vi "Get Attributes.vi"(8 "error in (no error)":errorcluster, 11 "For Loop Dialog in":refnum<class "Conditional Dialog.lvclass">) -> (0 "error out":errorcluster, 3 "For Loop Dialog out":refnum<class "Conditional Dialog.lvclass">)   [LabVIEW 2017, in "Conditional Dialog.lvclass"]
uses:
  Conditional Dialog.lvclass
  D:/Test-executive-builder/Source/Test Executive Builder Dialogs/ITest Executive Builder Dialog/ITest Executive Builder Dialog.lvclass
  ITest Executive Builder Dialog/ITest Executive Builder Dialog.lvclass/ITest Executive Builder Dialog.ctl
  Conditional Dialog.lvclass/Conditional Dialog.ctl
  210526c6-8347-4f83-98d4-bf6ff259764b.vi
  6281bc39-4b1f-4fa0-b6e5-3275a081bde5.vi
  37054371-845d-43d0-a581-1ea5269a3f09.vi
  <vilib>/Utility/error.llb/Clear Errors.vi
  <vilib>/gpm_packages/@cs/test-executive/Source/Test Executive/ITestExecutive/ITest Executive.lvclass
  Data Type Handler/Test Executive Builder Data Type Handler.lvclass
  ITest Executive Builder Dialog/ITest Executive Builder Dialog.lvclass
  <vilib>/gpm_packages/@cs/test-executive/Source/Test Executive/TestExecutive Ref/TestExecutive Ref.lvclass
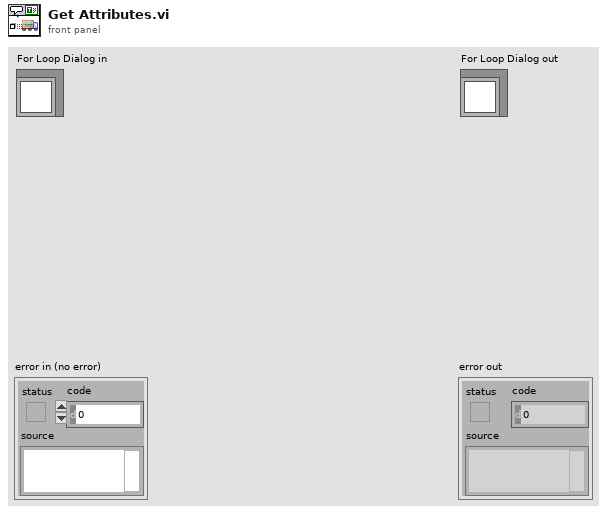
[diagram p1: front panel]
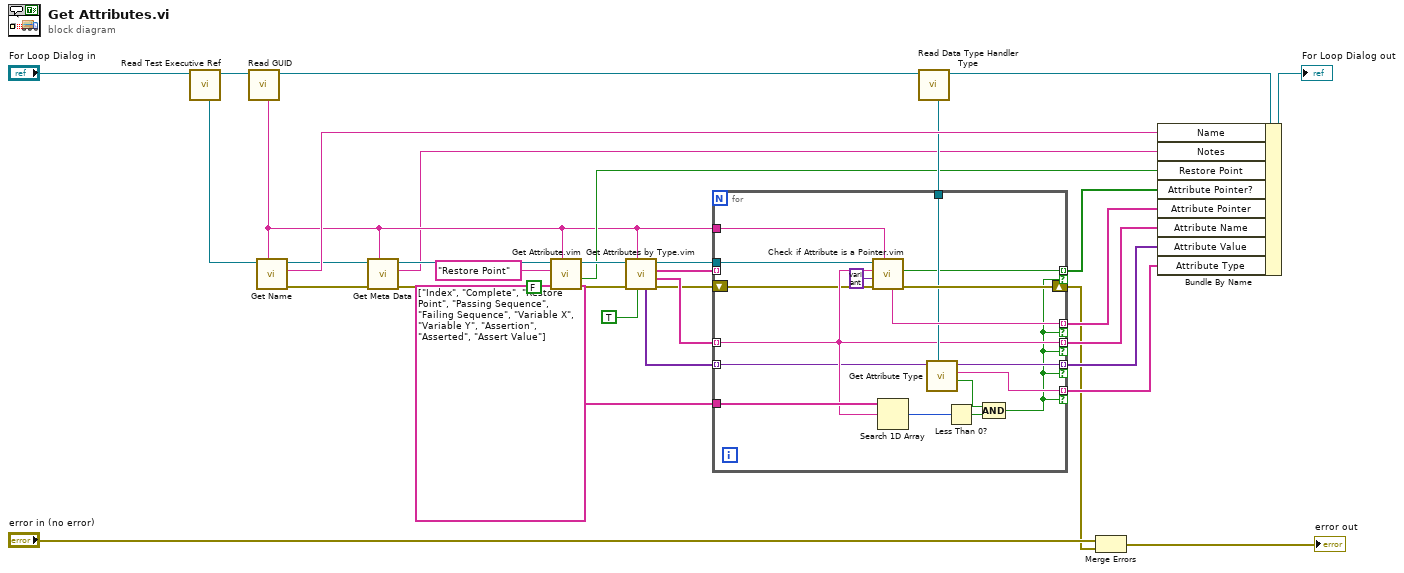
[diagram p0: block diagram]
diagram:
  n1 = call "Read Test Executive Ref.vi"("ITest Executive Builder Dialog in"="For Loop Dialog in") -> ("ITest Executive Builder Dialog out"=w33:refnum<class "Conditional Dialog.lvclass">, "Test Executive Ref"=w30:refnum<data-value>)  [unwired: 9 in]
  n2 = call "Read GUID.vi"("ITest Executive Builder Dialog in"=w33) -> ("ITest Executive Builder Dialog out"=w17:refnum<class "Conditional Dialog.lvclass">, "GUID"=w2:string)  [unwired: 9 in]
  n3 = call <vilib>:"Get Name.vi"("Unique ID"=w2, "Test Executive Ref"=w30) -> ("error out"=w4:errorcluster, "Name"=w32:string, "Test Executive Ref out"=w6:refnum<data-value>)  [unwired: 5 in, 2 out]
  n4 = call <vilib>:"Get Meta Data.vi"("Unique ID"=w2, "error in (no error)"=w4, "Test Executive Ref"=w6) -> ("error out"=w3:errorcluster, "Meta Data"=w1:string, "Test Executive Ref out"=w5:refnum<data-value>)  [unwired: 6 in]
  n5 = call "Get Attribute.vim"("ID"=w2, "error in (no error)"=w3, "Type"=FALSE, "Attribute Name"="Restore Point", "Test Executive Ref"=w5) -> ("error out"=w24:errorcluster, "Attribute"=w13:bool, "Test Executive Ref out"=w25:refnum<data-value>)  [unwired: 2 in, 2 out]
  n6 = call "Get Attributes by Type.vim"("Recurse Up List (Default=True)"=TRUE, "ID"=w2, "error in (no error)"=w24, "Test Executive Ref"=w25) -> ("error out"=w19:errorcluster, "Names"=w20:string[], "IDs"=w21:string[], "Test Executive Ref out"=w22:refnum<data-value>, "Attributes"=w18:variant[])  [unwired: 3 in]
  n7 = call "Read Data Type Handler Type.vi"("ITest Executive Builder Dialog in"=w17) -> ("ITest Executive Builder Dialog out"=w16:refnum<class "Conditional Dialog.lvclass">, "Data Type Handler"=w15:refnum<class "Test Executive Builder Data Type Handler.lvclass">)  [unwired: 9 in]
  n8 = for {
    tunnel: w22 -> [w37]
    tunnel: w21 -> [_] mode=indexing
    tunnel: w20 -> [w40] mode=indexing
    shift-right: [w50] -> w7
    shift-left: w19 -> [w36]
    tunnel: w2 -> [w41]
    tunnel: w18 -> [w39] mode=indexing
    tunnel: [w35] -> w12 mode=indexing if=w38
    tunnel: [w49] -> w11 mode=indexing if=w38
    tunnel: [w40] -> w10 mode=indexing if=w38
    tunnel: w15 -> [w48]
    tunnel: [w46] -> w8 mode=indexing if=w38
    tunnel: [w45] -> w9 mode=indexing if=w38
    tunnel: string[] ["Index", "Complete", "Restore Point", "Passing Sequence", "Failing Sequence", "Variable X", "Variable Y", "Assertion", "Asserted", "Assert Value"] -> [w44]
    n9 = call "Check if Attribute is a Pointer.vim"("ID"=w41, "error in (no error)"=w36, "Type"=variant, "Attribute Name"=w40, "Test Executive Ref"=w37) -> ("error out"=w50:errorcluster, "Pointer?"=w35:bool, "Pointer ID"=w49:string)  [unwired: 2 in, 2 out]
    n10 = Search 1D Array(1D array=w44, element=w40) -> (index of element=w43:i32)  [unwired: 1 in]
    n11 = call-dynamic "Get Attribute Type.vi"("Test Executive Builder Data Type Handler in"=w48, "Potential Attribute in"=w39) -> ("Valid Type?"=w47:bool, "Attribute Type"=w46:string, "Potential Attribute out"=w45:variant)  [unwired: 6 in, 1 out]
    n12 = Less Than 0?(x=w43) -> (x < 0?=w42:bool)
    n13 = Compound Arithmetic op=AND(w47, w42) -> (w38:bool)
  }
  n14 = Merge Errors("error in (no error)", w7) -> (→"error out":errorcluster)
  n15 = Bundle By Name(cluster=w16, "Name"=w32, "Notes"=w1, "Restore Point"=w13, "Attribute Pointer?"=w12, "Attribute Pointer"=w11, "Attribute Name"=w10, "Attribute Value"=w9, "Attribute Type"=w8) -> (→"For Loop Dialog out":refnum<class "Conditional Dialog.lvclass">)
